vi "xy_theta_to_transform.vi"(10 "Theta":dbl, 11 "XY":dbl[](array[numeric])) -> (3 "Transform matrix":T1)   [LabVIEW 2012]
uses:
  <vilib>/Analysis/Matrix/Datatypes/RealMatrix.ctl
  <vilib>/Analysis/Matrix/NI_Matrix.lvlib
panel:
  # "Turn XY and theta into a 2D (3x3) linear homogenous transform."
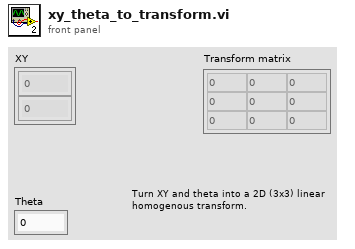
[diagram p1: front panel]
types:
  T1 = typedef "NI_Matrix.lvlib/RealMatrix.ctl" = dbl[][]
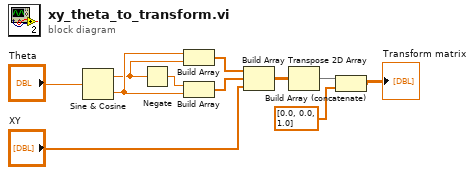
[diagram p0: block diagram]
diagram:
  n1 = Sine & Cosine(0:"Theta") -> (1:w2:dbl, 2:w4:dbl)
  n2 = Negate(x=w2) -> (-x=w3:dbl)
  n3 = Build Array(w4, w2) -> (w5:dbl[])
  n4 = Build Array(w3, w4) -> (w6:dbl[])
  n5 = Build Array(w5, w6, "XY") -> (w7:dbl[][])
  n6 = Transpose 2D Array(2D array=w7) -> (transposed array=w8:dbl[][])
  n7 = Build Array (concatenate)(w8, dbl[] [0.0, 0.0, 1.0] ("array w/ subset deleted")) -> (→"Transform matrix":dbl[][])
